vi "Launcher.vi"() -> ()   [LabVIEW 2016]
doc: "Use this template to build a user interface event handler design pattern. Use this pattern for dialog boxes and other user interfaces. You also can create and execute user-defined events that the VI can handle the same way as user interface events."
uses:
  Classes/Rectangle Mask/Rectangle Mask.lvclass
  <vilib>/Utility/miscctls.llb/LVRectTypeDef.ctl
panel:
  in  "Highlight Control 2":bool
  in  "Highlight Control":bool
  in  "Highlight Panel":bool
  in  "stop":bool
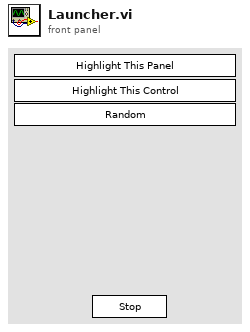
[diagram p1: front panel]
types:
  T1 = typedef "LVRectTypeDef.ctl" = cluster{"Left":i16, "Top":i16, "Right":i16, "Bottom":i16}
  T2 = typedef "LVPointTypeDef.ctl" = cluster{"Horizontal":i16, "Vertical":i16}
  T3 = typedef "LVPositionTypeDef.ctl" = cluster{"Left":i32, "Top":i32}
  T4 = typedef "LVBoundsTypeDef.ctl" = cluster{"Width":u32, "Height":u32}
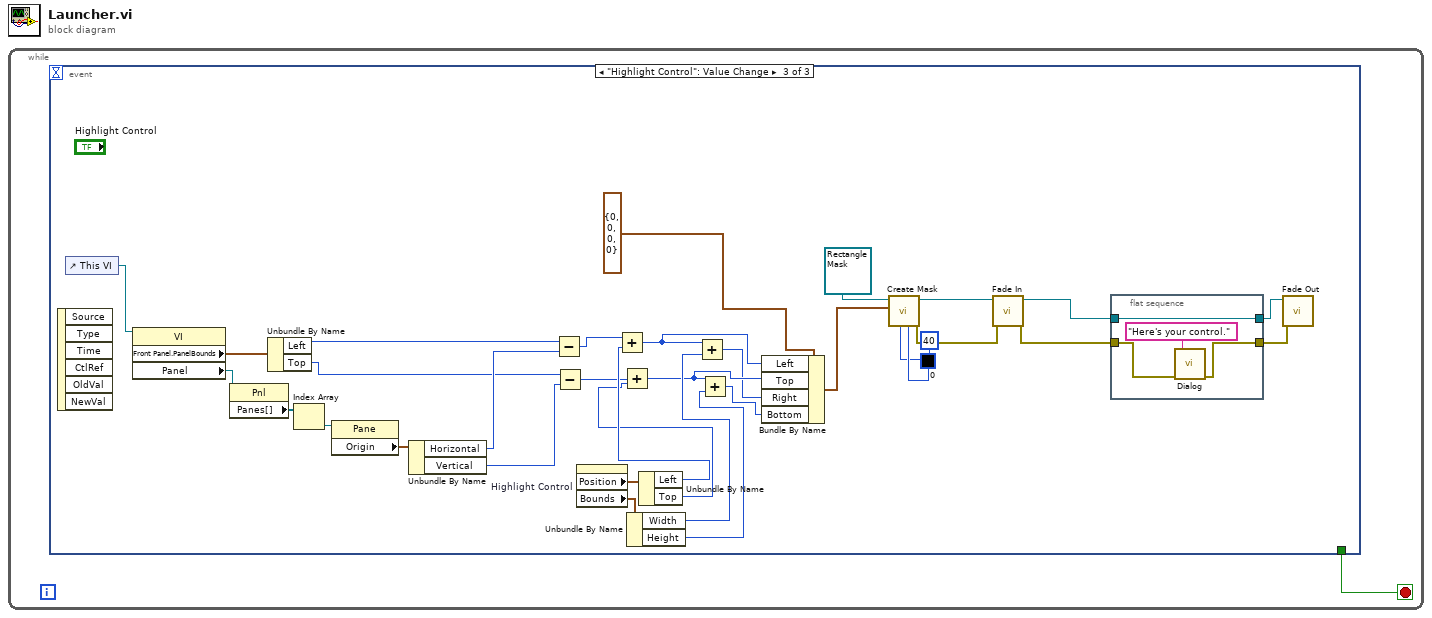
[diagram p0: block diagram]
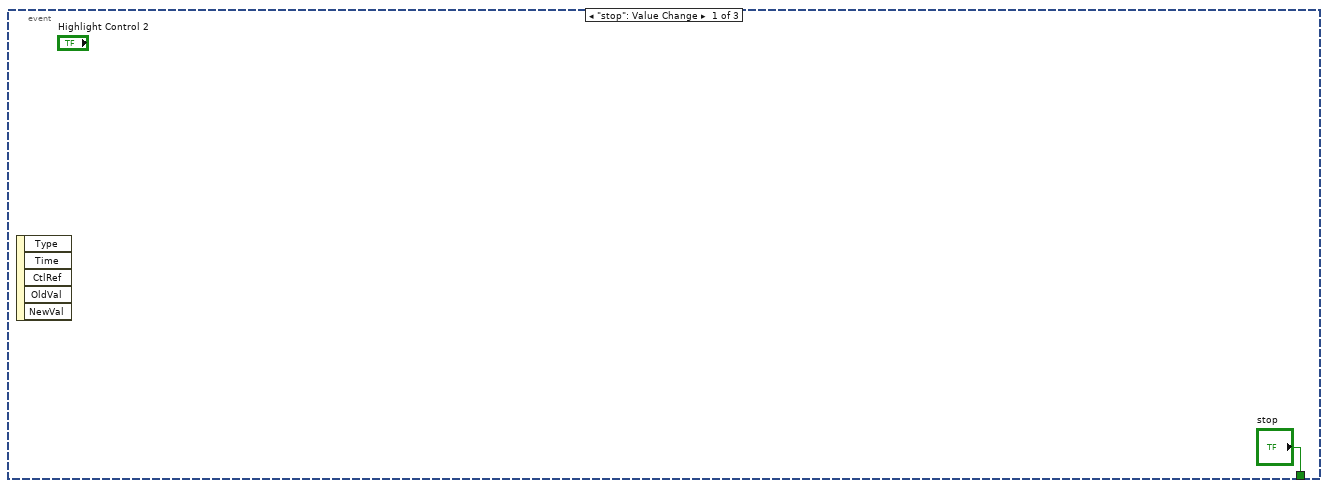
[diagram p2: hidden frame]
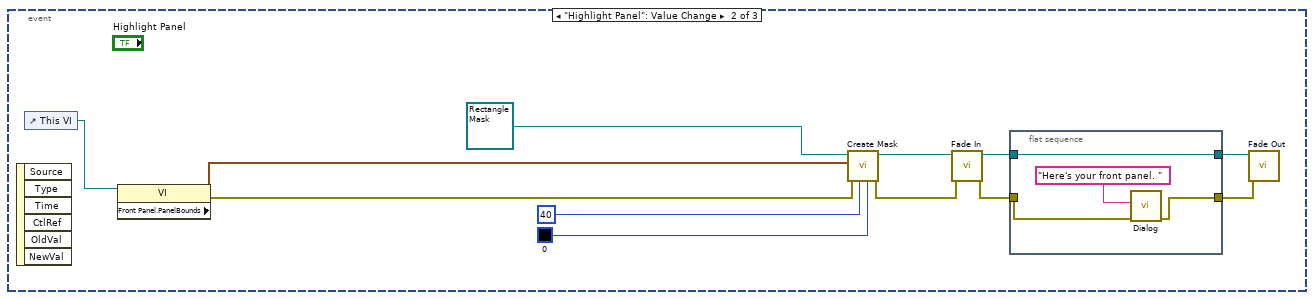
[diagram p3: hidden frame]
diagram:
  n1 = while {
    stop <- w1 stop-if-true
    n2 = event shown="[2] \"Highlight Control\": Value Change" {
      selector: _ -> [_ _ _]
      dyn-events: _ -> [_ _ _]
      timeout: _ -> [_ _ _]
      tunnel: ["stop" _ _] -> w1
      event "stop": Value Change {
        n3 = event-data() -> ()  [unwired: 1 in, 5 out]
      }
      event "Highlight Panel": Value Change {
        n4 = event-data() -> ()  [unwired: 1 in, 6 out]
        n5 = control-ref of="This VI"() -> (w5:refnum<vi>)
        n6 = property class="VI"(reference=w5) -> (error out=w6:errorcluster, "Front Panel.PanelBounds"=w14:T1)  [unwired: 1 in, 1 out]
        n7 = call-dynamic "Create Mask.vi"("Color"=u32 0, "Transparency"=u8 40, "Error in"=w6, "Bounds"=w14, "Rectangle Mask In"=refnum<class "Rectangle Mask.lvclass"> refnum ("Rectangle Mask.lvclass")) -> ("Error out"=w10:errorcluster, "Rectangle Mask Out"=w9:refnum<class "Rectangle Mask.lvclass">)  [unwired: 5 in]
        n8 = call-dynamic "Fade In.vi"("error in (no error)"=w10, "Rectangle Mask in"=w9) -> ("error out"=w12:errorcluster, "Rectangle Mask out"=w11:refnum<class "Rectangle Mask.lvclass">)  [unwired: 8 in]
        n9 = flat-sequence {
          tunnel: w11 -> [w18]
          tunnel: [w18] -> w4
          tunnel: w12 -> [w17]
          tunnel: [w16] -> w3
          frame #0 {
            n10 = call "Dialog.vi"("Error in"=w17, "message"="Here's your front panel. ") -> ("Error out"=w16:errorcluster)  [unwired: 9 in]
          }
        }
        n11 = call-dynamic "Fade Out.vi"("error in (no error)"=w3, "Rectangle Mask in"=w4) -> ()  [unwired: 8 in, 2 out]
      }
      event "Highlight Control": Value Change {
        n12 = event-data() -> ()  [unwired: 1 in, 6 out]
        n13 = control-ref of="This VI"() -> (w44:refnum<vi>)
        n14 = property class="VI"(reference=w44) -> ("Front Panel.PanelBounds"=w39:T1, "Panel"=w43:refnum<vi>)  [unwired: 1 in, 2 out]
        n15 = property class="Pnl"(reference=w43) -> ("Panes[]"=w42:refnum<vi>[])  [unwired: 1 in, 2 out]
        n16 = Unbundle By Name(w39) -> ("Left"=w38:i16, "Top"=w36:i16)
        n17 = Index Array(array=w42) -> (element=w41:refnum<vi>)  [unwired: 1 in]
        n18 = property class="Pane"(reference=w41) -> ("Origin"=w40:T2)  [unwired: 1 in, 2 out]
        n19 = Unbundle By Name(w40) -> ("Horizontal"=w37:i16, "Vertical"=w35:i16)
        n20 = Subtract(x=w38, y=w37) -> (x-y=w34:i16)
        n21 = Subtract(x=w36, y=w35) -> (x-y=w31:i16)
        n22 = property on="Highlight Control" class="Bool"() -> ("Position"=w33:T3, "Bounds"=w29:T4)  [unwired: 2 in, 2 out]
        n23 = Unbundle By Name(w29) -> ("Width"=w28:u32, "Height"=w27:u32)
        n24 = Unbundle By Name(w33) -> ("Left"=w32:i32, "Top"=w30:i32)
        n25 = Add(x=w34, y=w32) -> (x+y=w25:i32)
        n26 = Add(x=w31, y=w30) -> (x+y=w24:i32)
        n27 = Add(x=w25, y=w28) -> (x+y=w23:u32)
        n28 = Add(x=w24, y=w27) -> (x+y=w22:u32)
        n29 = Bundle By Name(cluster=T1 {"Left"=0, "Top"=0, "Right"=0, "Bottom"=0} ("Bounds"), "Left"=w25, "Top"=w24, "Right"=w23, "Bottom"=w22) -> (w21:T1)
        n30 = call-dynamic "Create Mask.vi"("Color"=u32 0, "Transparency"=u8 40, "Bounds"=w21, "Rectangle Mask In"=refnum<class "Rectangle Mask.lvclass"> refnum ("Rectangle Mask.lvclass")) -> ("Error out"=w48:errorcluster, "Rectangle Mask Out"=w47:refnum<class "Rectangle Mask.lvclass">)  [unwired: 6 in]
        n31 = call-dynamic "Fade In.vi"("error in (no error)"=w48, "Rectangle Mask in"=w47) -> ("error out"=w50:errorcluster, "Rectangle Mask out"=w49:refnum<class "Rectangle Mask.lvclass">)  [unwired: 8 in]
        n32 = flat-sequence {
          tunnel: w49 -> [w53]
          tunnel: [w53] -> w20
          tunnel: w50 -> [w55]
          tunnel: [w54] -> w19
          frame #0 {
            n33 = call "Dialog.vi"("Error in"=w55, "message"="Here's your control.") -> ("Error out"=w54:errorcluster)  [unwired: 9 in]
          }
        }
        n34 = call-dynamic "Fade Out.vi"("error in (no error)"=w19, "Rectangle Mask in"=w20) -> ()  [unwired: 8 in, 2 out]
      }
    }
  }
